vi "Lookahead.vi"(8 "error in (no error)":errorcluster, 10 "Offset past next":i32, 11 "Alpaca Parser in":refnum<class "Parser.lvclass">) -> (0 "error out":errorcluster, 1 "Lookahead Value":string, 2 "Lookahead Type":i32, 3 "Alpaca Parser out":refnum<class "Parser.lvclass">)   [LabVIEW 2013, in "JKI JSON Serialization.lvlib" / "Parser.lvclass"]
uses:
  Parser.lvclass
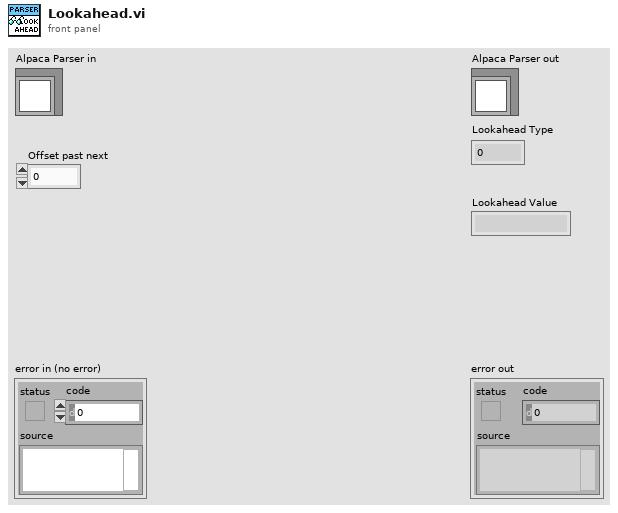
[diagram p1: front panel]
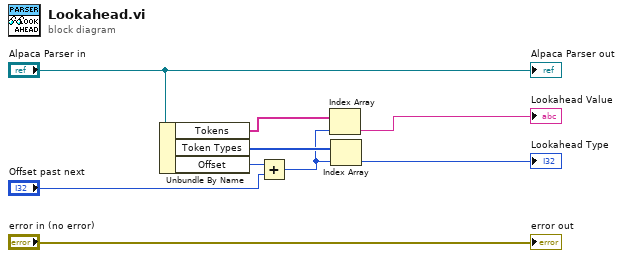
[diagram p0: block diagram]
diagram:
  n1 = Unbundle By Name("Alpaca Parser in") -> ("Tokens"=w4:string[], "Token Types"=w5:i32[], "Offset"=w3:i32)
  n2 = Add(x=w3, y="Offset past next") -> (x+y=w2:i32)
  n3 = Index Array(array=w4, index=w2) -> (element=→"Lookahead Value":string)
  n4 = Index Array(array=w5, index=w2) -> (element=→"Lookahead Type":i32)
  "error out" <- "error in (no error)"
  "Alpaca Parser out" <- "Alpaca Parser in"
